vi "Enumerate.vi"(8 "error in (no error)":errorcluster, 11 "IP Connection in":refnum<class "IP Connection.lvclass">) -> (0 "error out":errorcluster, 3 "IP Connection out":refnum<class "IP Connection.lvclass">)   [LabVIEW 2011, in "Tinkerforge.lvlib" / "IP Connection.lvclass"]
doc: "This VI sends an enumerate message to the stack. The package contains no payload and is sended to stack ID 0 (broadcast). There is no direct response to this package."
uses:
  IP Connection.lvclass
  Type Definitions/Functions.ctl
  IP Connection.lvclass/IP Connection.ctl
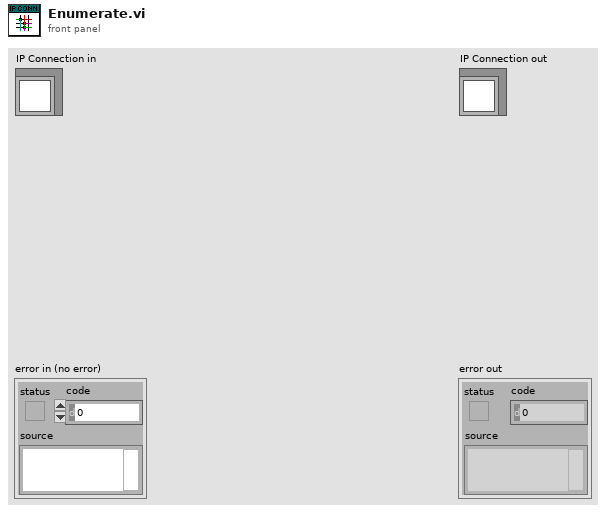
[diagram p1: front panel]
types:
  T1 = typedef "Tinkerforge.lvlib/IP Connection.lvclass/Functions.ctl" = enum8{"no Global Function", "get stack id", "enumerate", "CB enumerate"}
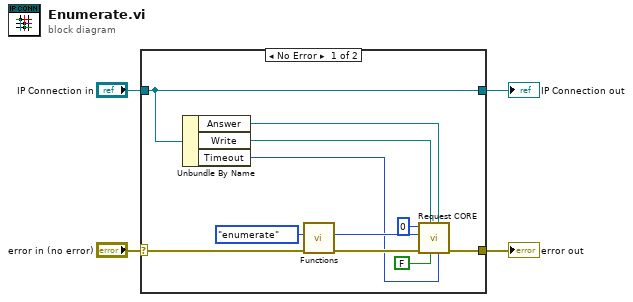
[diagram p0: block diagram]
diagram:
  n1 = case shown="No Error" "error in (no error)" {
    selector: "error in (no error)" -> [w15 w17]
    tunnel: [w7 w17] -> w3
    tunnel: [w13 w16] -> w1
    tunnel: "IP Connection in" -> [w13 w16]
    frame No Error {
      n2 = Unbundle By Name(w13) -> ("Answer"=w8:refnum<user-event>, "Write"=w9:refnum<queue>, "Timeout"=w6:i32)
      n3 = call "Functions.vi"("Error In"=w15, "Function in"=Functions."enumerate") -> ("Error Out"=w12:errorcluster, "Function ID out"=w11:u8)  [unwired: 7 in, 1 out]
      n4 = call "Request CORE.vi"("Timeout"=w6, "Answer UE"=w8, "Response"=FALSE, "Write"=w9, "Error In"=w12, "Function ID"=w11, "Stack ID"=u8 0) -> ("Error Out"=w7:errorcluster)  [unwired: 1 in, 3 out]
    }
    frame Error {
    }
  }
  "error out" <- w3
  "IP Connection out" <- w1
